vi "CSM - Keywords.vi"() -> (2 "Keywords (%Hex Format)":string[](array[string]), 3 "Keywords":string[](array[string]))   [LabVIEW 2017, in "Communicable State Machine.lvlib"]
doc: "Lists keywords in CSM messages and their %Hex format.\n\n> [!NOTE] <b>CSM Message Keywords</b>\n>\n> The following are CSM message keywords: `->`, `->|`, `-@`, `-&`, `<-`, `\\r`, `\\n`, `//`, `>>`, `>>>`, `>>>`, `;`, `,`.\n\n\n-- <b>Indicators</b> --\n- <b>keywords</b>: List of CSM keywords.\n- <b>Keywords (%Hex Format)</b>: The %Hex format of the CSM keyword list."
uses:
  Communicable State Machine.lvlib
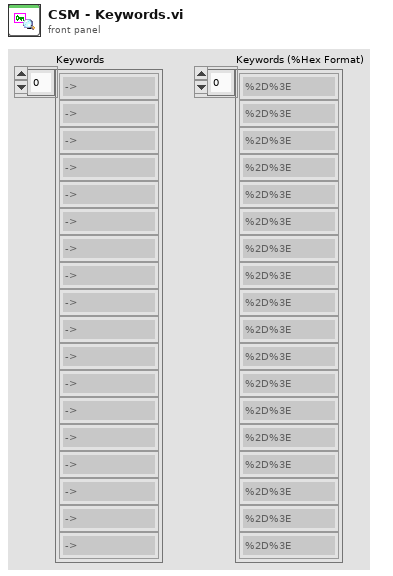
[diagram p1: front panel]
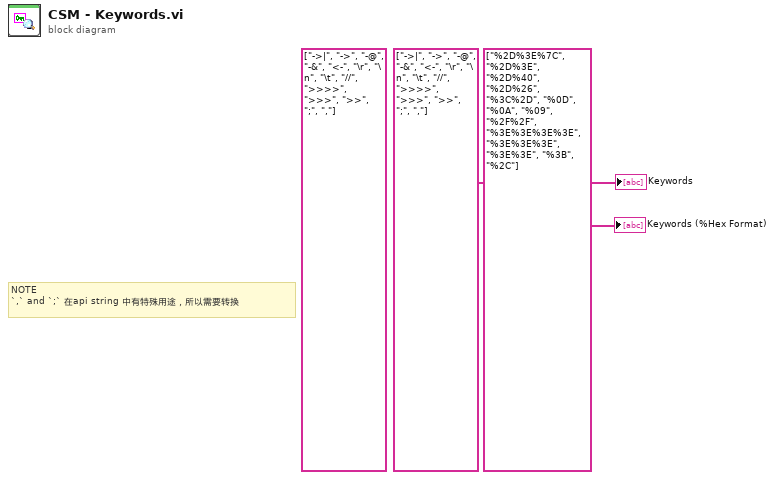
[diagram p0: block diagram]
diagram:
  (unwired) string[] ["->|", "->", "-@", "-&", "<-", "\r", "\n", "\t", "//", ">>>>", ">>>", ">>", ";", ","]
  # "NOTE\n`,` and `;` 在api string 中有特殊用途，所以需要转换"
  "Keywords (%Hex Format)" <- string[] ["%2D%3E%7C", "%2D%3E", "%2D%40", "%2D%26", "%3C%2D", "%0D", "%0A", "%09", "%2F%2F", "%3E%3E%3E%3E", "%3E%3E%3E", "%3E%3E", "%3B", "%2C"]
  "Keywords" <- string[] ["->|", "->", "-@", "-&", "<-", "\r", "\n", "\t", "//", ">>>>", ">>>", ">>", ";", ","]
